vi "布线第一个点放到甩线前最后一点.vi"(10 "布线点":string[](array[string]), 11 "甩线前":string[](array[string])) -> (2 "布线点 2":string[](array[string]), 3 "甩线前 2":string[](array[string]))   [LabVIEW 2014]
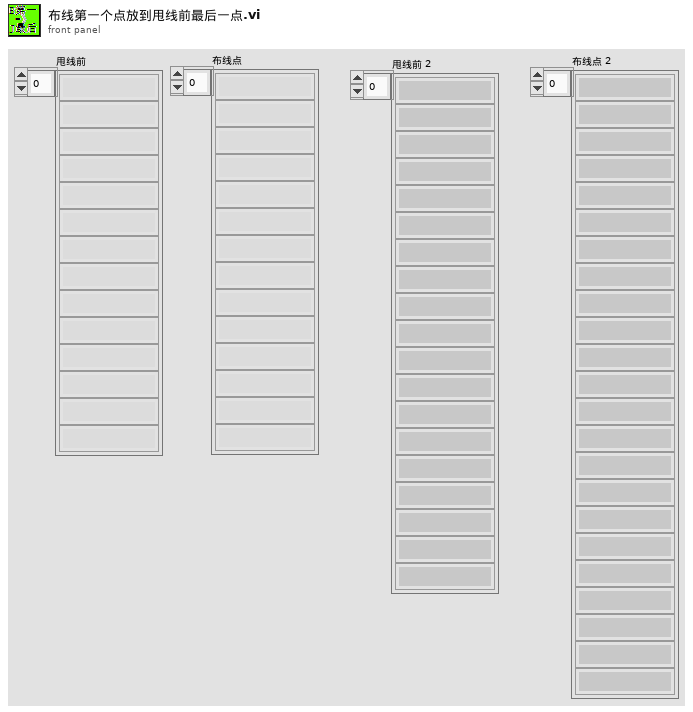
[diagram p1: front panel]
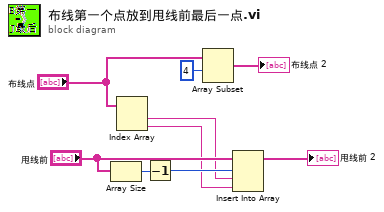
[diagram p0: block diagram]
diagram:
  n1 = Array Size(array="甩线前") -> (size(s)=w8:i32)
  n2 = Index Array(array="布线点") -> (element #1=w2:string, element #2=w1:string)  [unwired: 2 in]
  n3 = Decrement(x=w8) -> (x-1=w7:i32)
  n4 = Array Subset(array="布线点", index=4 ("索引")) -> (→"布线点 2":string[])  [unwired: 1 in]
  n5 = Insert Into Array(array="甩线前", index=w7, new element #1=w2, new element #2=w1) -> (→"甩线前 2":string[])
